vi "Left Encoder Read.vi"() -> (0 "Stopped":bool, 1 "Direction":bool, 2 "Rate":dbl, 3 "Distance":dbl, 4 "Ave Velocity":dbl)   [LabVIEW 2015]
uses:
  Support/Global Objects.vi
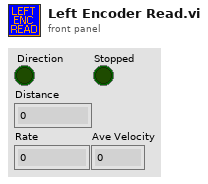
[diagram p1: front panel]
types:
  T1 = typedef "Encoder Info.ctl" = cluster{"EncoderDevRef":T2, "Velocity Samples":dbl[], "Velocity Index":u32}
  T2 = typedef "WPI_EncoderDevRef.ctl" = cluster{"DevStatus":errorcluster, "EncoderIndex":T3, "CounterIndex":T4, "DistancePerCount":dbl, "Decoding Type":T5}
  T3 = typedef "FPGA_EncoderIdx.ctl" = enum8{"Enc 0", "Enc 1", "Enc 2", "Enc 3", "Enc 4", "Enc 5", "Enc 6", "Enc 7", "Invalid"}
  T4 = typedef "FPGA_CounterCtrSystemIndex.ctl" = enum8{"Ctr 0", "Ctr 1", "Ctr 2", "Ctr 3", "Ctr 4", "Ctr 5", "Ctr 6", "Ctr 7", "Invalid"}
  T5 = typedef "WPI_EncoderType.ctl" = enum16{"1x", "2x", "4x"}
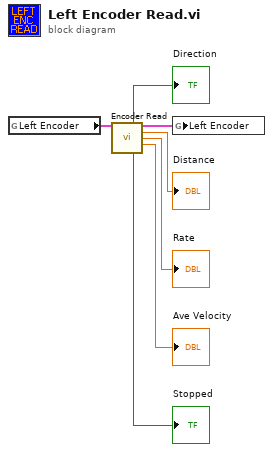
[diagram p0: block diagram]
diagram:
  n1 = global read "Global Objects.vi" "Left Encoder"() -> (w7:T1)
  n2 = call "Encoder Read.vi"("Encoder Info"=w7) -> ("Direction"=→"Direction":bool, "Encoder Out"=w2:T1, "Distance"=→"Distance":dbl, "Rate"=→"Rate":dbl, "Ave Velocity"=→"Ave Velocity":dbl, "Stopped"=→"Stopped":bool)  [unwired: 8 in, 1 out]
  n3 = global write "Global Objects.vi" "Left Encoder"(w2) -> ()
